vi "panel_update_status_string.vi"(8 "error in (no error)":errorcluster, 10 "String":string, 11 "galvo_panel in":refnum<class "galvo_panel.lvclass">) -> (0 "error out":errorcluster, 3 "galvo_panel out":refnum<class "galvo_panel.lvclass">)   [LabVIEW 2015, in "galvo_panel.lvclass"]
uses:
  galvo_panel.lvclass
  galvo_panel.lvclass/galvo_panel.ctl
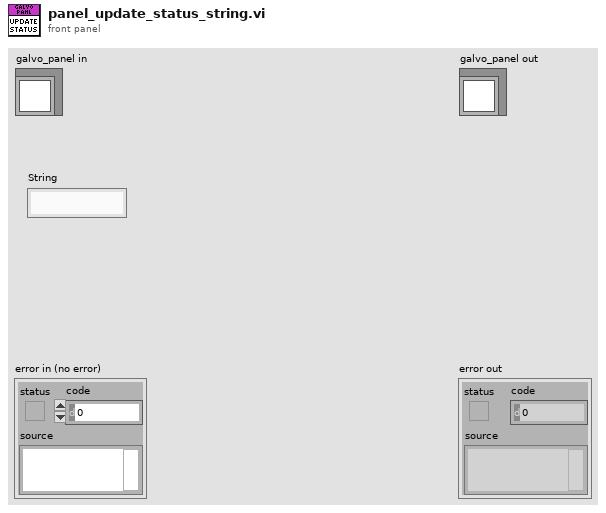
[diagram p1: front panel]
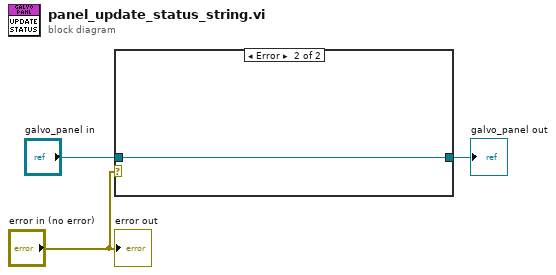
[diagram p0: block diagram]
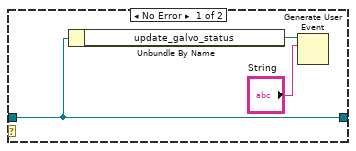
[diagram p2: hidden frame]
diagram:
  n1 = case shown="Error" "error in (no error)" {
    tunnel: "galvo_panel in" -> [w4 w7]
    tunnel: [w4 w7] -> w1
    frame No Error {
      n2 = Unbundle By Name(w4) -> ("update_galvo_status"=w6:refnum<user-event>)
      n3 = Generate User Event(user event=w6, event data cluster="String") -> ()  [unwired: 2 in, 2 out]
    }
    frame Error {
    }
  }
  "galvo_panel out" <- w1
  "error out" <- "error in (no error)"
